vi "PreChirper apply prism values.vi"(8 "error in (no error)":errorcluster, 11 "Wavelength":dbl) -> (0 "error out":errorcluster)   [LabVIEW 2017]
uses:
  Prechirper commands.ctl
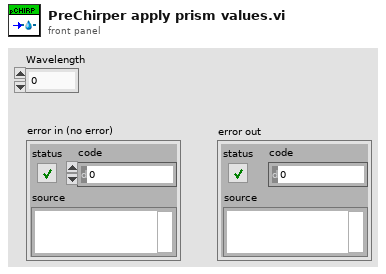
[diagram p1: front panel]
types:
  T1 = typedef "Prechirper commands.ctl" = enum16{"Prism 1 read", "Prism 1 set", "Prism 2 read", "Prism 2 set", "Wavelength read", "Wavelength Femto set", "Wavelength Femto and Laser set", "GVD curve number read", "GVD curve number set"}
  T2 = enum16{"Initialise", "Load from file", "Save to file", "Read", "Write"}
  T3 = typedef "Calibration config.ctl" = cluster{"Current Objective":string, "Objective Settings":T4[], "PreChirper Values Preset ?":bool, "PreChirper Settings":T5[], "PreChirper Constants":T6}
  T4 = typedef "Objective Config.ctl" = cluster{"Name":string, "Sum X":dbl, "Sum Y":dbl, "Diff X":dbl, "Diff Y":dbl, "Distortion Correction":dbl, "Z_norm to um_scaling":dbl, "X_norm to um_scaling":dbl, "Calibrated Wavelength":dbl}
  T5 = typedef "Prechirper Cal Config.ctl" = cluster{"Wavelength":i32, "Prism 1":i32, "Prism 2":i32}
  T6 = typedef "PreChirper constants.ctl" = cluster{"a 1":i32, "b 1":i32, "c 1":i32, "a 2":i32, "b 2":i32, "c 2":i32, "lmin":i32, "lmax":i32}
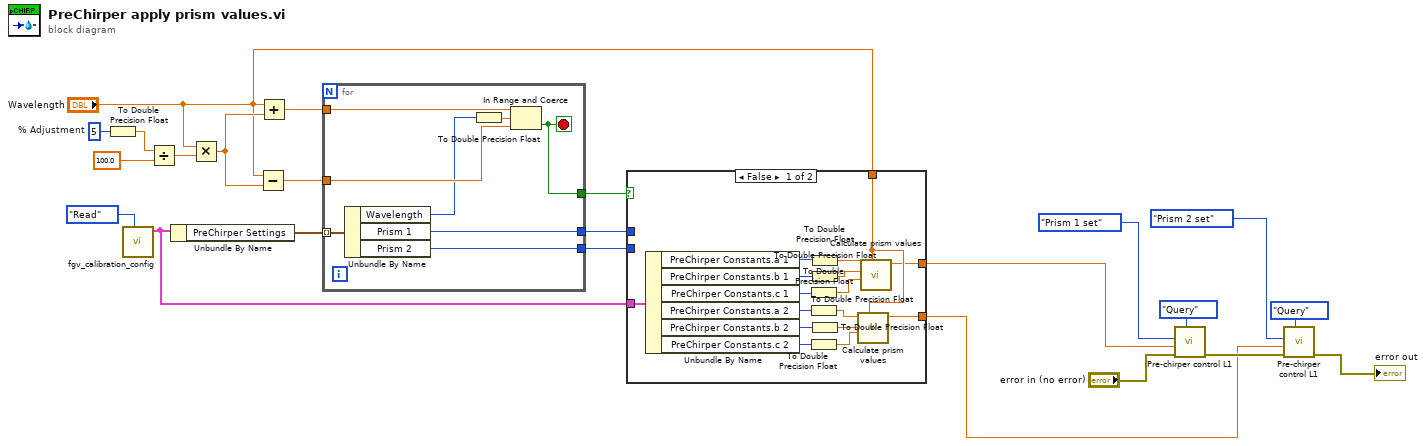
[diagram p0: block diagram]
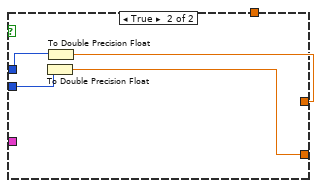
[diagram p2: hidden frame]
diagram:
  w21 = 5  # % Adjustment
  n1 = To Double Precision Float(number=w21) -> (double precision float=w20:dbl)
  n2 = call "fgv_calibration_config.vi"("Cal config ops"=T2."Read") -> ("Config cluster OUT"=w6:T3)  [unwired: 9 in, 1 out]
  n3 = Divide(x=w20, y=100.0) -> (x/y=w18:dbl)
  n4 = Unbundle By Name(w6) -> ("PreChirper Settings"=w22:T5[])
  n5 = Multiply(x="Wavelength", y=w18) -> (x*y=w17:dbl)
  n6 = Subtract(x="Wavelength", y=w17) -> (x-y=w16:dbl)
  n7 = Add(x="Wavelength", y=w17) -> (x+y=w15:dbl)
  n8 = for {
    tunnel: w22 -> [w31] mode=indexing
    tunnel: w16 -> [w29]
    tunnel: w15 -> [w30]
    tunnel: [w26] -> w12
    tunnel: [w25] -> w13
    tunnel: [w24] -> w14
    stop <- w24 stop-if-true
    n9 = Unbundle By Name(w31) -> ("Wavelength"=w27:i32, "Prism 1"=w26:i32, "Prism 2"=w25:i32)
    n10 = To Double Precision Float(number=w27) -> (double precision float=w28:dbl)
    n11 = In Range and Coerce(upper limit=w30, x=w28, lower limit=w29) -> (In Range?=w24:bool)  [unwired: 1 out]
  }
  n12 = case shown="False" w14 {
    tunnel: w13 -> [_ w50]
    tunnel: w12 -> [_ w51]
    tunnel: w6 -> [w47 _]
    tunnel: "Wavelength" -> [w46 _]
    tunnel: [w33 w48] -> w3
    tunnel: [w32 w49] -> w4
    frame False {
      n13 = Unbundle By Name(w47) -> ("PreChirper Constants.a 1"=w45:i32, "PreChirper Constants.b 1"=w44:i32, "PreChirper Constants.c 1"=w43:i32, "PreChirper Constants.a 2"=w39:i32, "PreChirper Constants.b 2"=w38:i32, "PreChirper Constants.c 2"=w37:i32)
      n14 = To Double Precision Float(number=w43) -> (double precision float=w40:dbl)
      n15 = To Double Precision Float(number=w39) -> (double precision float=w36:dbl)
      n16 = To Double Precision Float(number=w37) -> (double precision float=w34:dbl)
      n17 = To Double Precision Float(number=w45) -> (double precision float=w42:dbl)
      n18 = To Double Precision Float(number=w44) -> (double precision float=w41:dbl)
      n19 = To Double Precision Float(number=w38) -> (double precision float=w35:dbl)
      n20 = call "Calculate prism values.vi"("wavelength"=w46, "c"=w34, "b"=w35, "a"=w36) -> ("prism value"=w33:dbl)  [unwired: 7 in]
      n21 = call "Calculate prism values.vi"("wavelength"=w46, "c"=w40, "b"=w41, "a"=w42) -> ("prism value"=w32:dbl)  [unwired: 7 in]
    }
    frame True {
      n22 = To Double Precision Float(number=w50) -> (double precision float=w48:dbl)
      n23 = To Double Precision Float(number=w51) -> (double precision float=w49:dbl)
    }
  }
  n24 = call "Pre-chirper control L1.vi"("State"=enum16{"Initialise", "Query", "Close"}."Query", "error in (no error)"="error in (no error)", "Data to Set"=w4, "Pre-chirper commands"=Prechirper_commands."Prism 1 set") -> ("error out"=w9:errorcluster)  [unwired: 6 in, 1 out]
  n25 = call "Pre-chirper control L1.vi"("State"=enum16{"Initialise", "Query", "Close"}."Query", "error in (no error)"=w9, "Data to Set"=w3, "Pre-chirper commands"=Prechirper_commands."Prism 2 set") -> ("error out"=→"error out":errorcluster)  [unwired: 6 in, 1 out]
